vi "replaceDateToken.vi"(8 "error in (no error)":errorcluster, 10 "Query In":string, 11 "Transaction in":refnum<class "Transaction.lvclass">) -> (0 "error out":errorcluster, 2 "Query Out":string, 3 "Transaction out":refnum<class "Transaction.lvclass">)   [LabVIEW 2018, in "Transaction.lvclass"]
uses:
  Transaction.lvclass
  Transaction.lvclass/Transaction.ctl
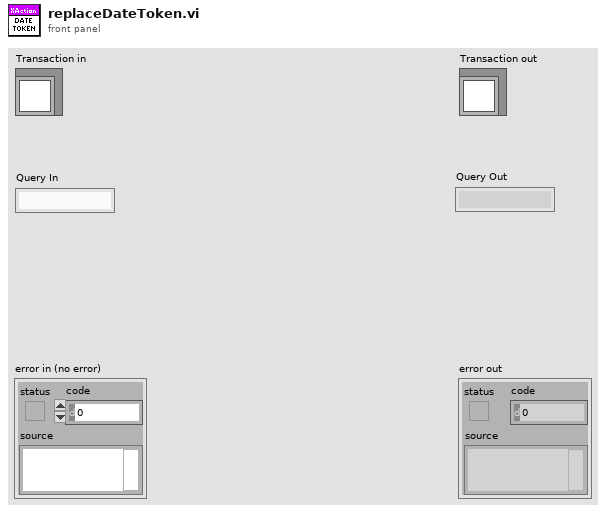
[diagram p1: front panel]
types:
  T1 = typedef "LVDateTimeRec.ctl" = cluster{"fractional second":dbl, "second":i32, "minute":i32, "hour":i32, "day of month":i32, "month":i32, "year":i32, "day of week":i32, "day of year":i32, "DST":i32}
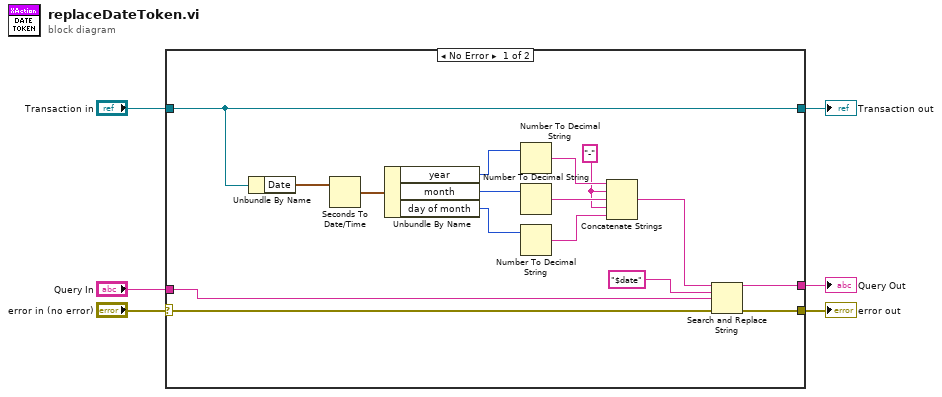
[diagram p0: block diagram]
diagram:
  n1 = case shown="No Error" "error in (no error)" {
    selector: "error in (no error)" -> [w12 w24]
    tunnel: [w11 w24] -> w5
    tunnel: [w22 w23] -> w3
    tunnel: "Transaction in" -> [w22 w23]
    tunnel: "Query In" -> [w8 _]
    tunnel: [w9 _] -> w1
    frame No Error {
      w18 = "-"
      n2 = Unbundle By Name(w22) -> ("Date"=w13:timestamp)
      n3 = Seconds To Date/Time(time stamp (now)=w13) -> (date time rec=w14:T1)  [unwired: 1 in]
      n4 = Unbundle By Name(w14) -> ("year"=w15:i32, "month"=w16:i32, "day of month"=w17:i32)
      n5 = Number To Decimal String(number=w15) -> (decimal integer string=w19:string)  [unwired: 1 in]
      n6 = Number To Decimal String(number=w16) -> (decimal integer string=w20:string)  [unwired: 1 in]
      n7 = Number To Decimal String(number=w17) -> (decimal integer string=w21:string)  [unwired: 1 in]
      n8 = Concatenate Strings(w19, w18, w20, w18, w21) -> (w10:string)
      n9 = Search and Replace String(input string=w10, search string="$date", replace string=w8, error in=w12) -> (result string=w9:string, error out=w11:errorcluster)  [unwired: 4 in, 2 out]
    }
    frame Error {
    }
  }
  "error out" <- w5
  "Transaction out" <- w3
  "Query Out" <- w1
